vi "SimpleInterface.vi"() -> ()   [LabVIEW 2015]
panel:
  out "Amplitud\nP100":dbl
  out "N75":dbl
  out "P100":dbl
  out "N145":dbl
  out "Latencia \npromedio":dbl
  out "Resultado de las pruebas":cluster{dbl[], dbl[]}[](graph)
  in  "Cantidad de\nestímulos":dbl
  in  "Comenzar \nprueba":bool
  in  "Cantidad de \ncuadros":dbl
  in  "stop":bool
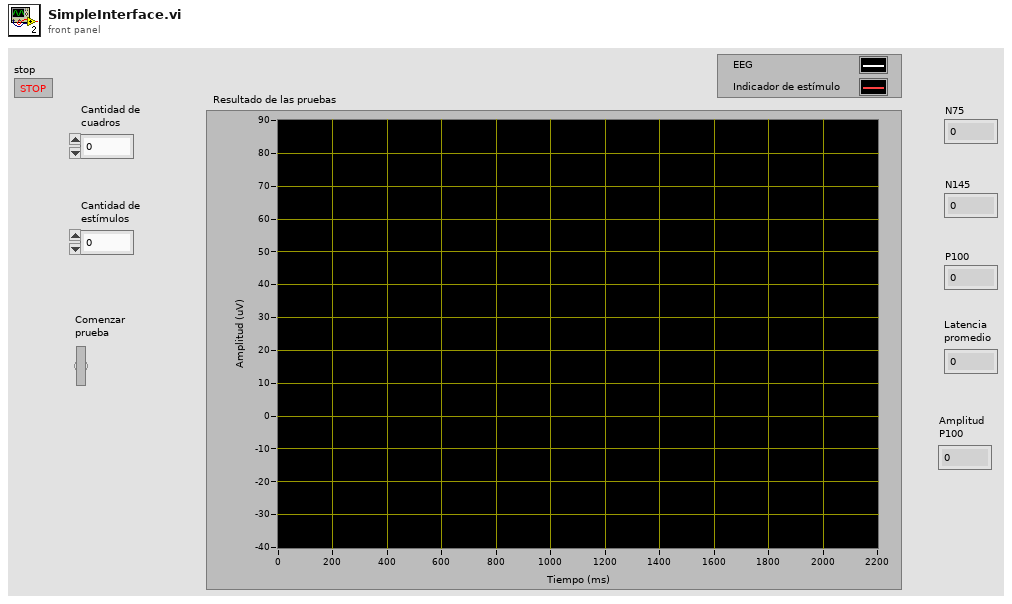
[diagram p1: front panel]
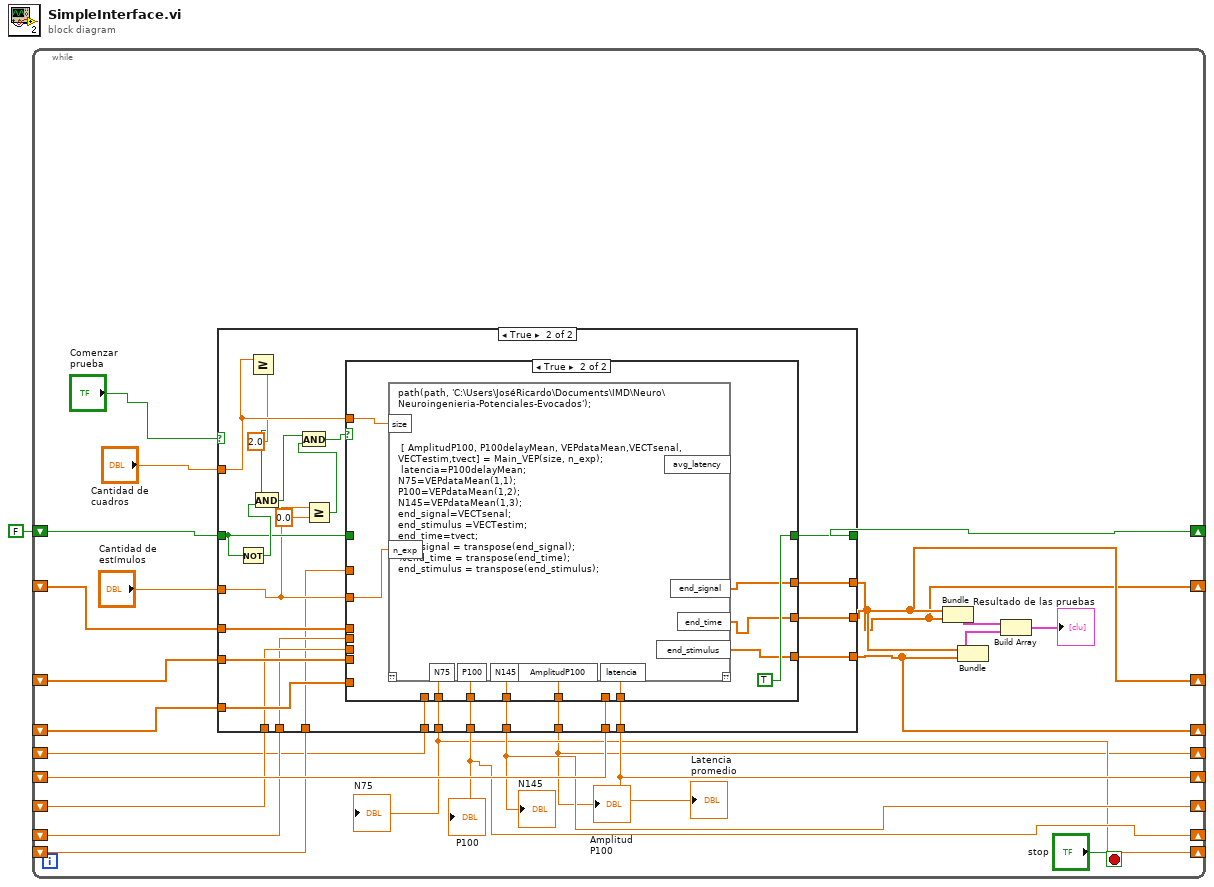
[diagram p0: block diagram]
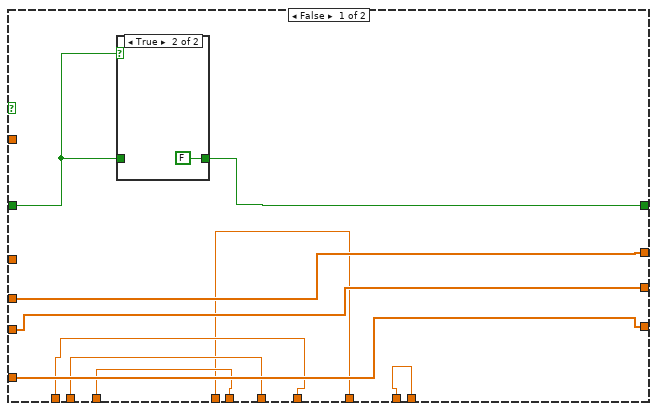
[diagram p2: hidden frame]
diagram:
  n1 = while {
    shift-right: [w25] -> _
    shift-left: FALSE -> [w23]
    shift-right: [w17] -> _
    shift-left: _ -> [w13]
    shift-right: [w16] -> _
    shift-left: _ -> [w14]
    shift-right: [w15] -> _
    shift-left: _ -> [w12]
    shift-right: [w11] -> _
    shift-left: _ -> [w10]
    shift-right: [w9] -> _
    shift-left: _ -> [w6]
    shift-right: [w8] -> _
    shift-left: _ -> [w5]
    shift-right: [w7] -> _
    shift-left: _ -> [w4]
    shift-right: [w3] -> _
    shift-left: _ -> [w2]
    stop <- "stop" stop-if-true
    n2 = case shown="True" "Comenzar \nprueba" {
      tunnel: [w36 w61] -> w25
      tunnel: "Cantidad de \ncuadros" -> [_ w65]
      tunnel: w23 -> [w35 w60]
      tunnel: "Cantidad de\nestímulos" -> [_ w59]
      tunnel: [w33 w54] -> w17
      tunnel: [w32 w53] -> w15
      tunnel: [w34 w52] -> w16
      tunnel: w14 -> [w34 w51]
      tunnel: w13 -> [w33 w50]
      tunnel: w12 -> [w32 w49]
      tunnel: [w31 w48] -> w11
      tunnel: w10 -> [w31 w47]
      tunnel: [w30 w46] -> w9
      tunnel: [w29 w45] -> w8
      tunnel: [w28 w44] -> w7
      tunnel: w6 -> [w30 w43]
      tunnel: w5 -> [w29 w42]
      tunnel: w4 -> [w28 w41]
      tunnel: [w27 w40] -> w3
      tunnel: w2 -> [w27 w39]
      frame False {
        n3 = case shown="True" w35 {
          tunnel: [w37 FALSE] -> w36
          tunnel: w35 -> [w37 _]
          frame False {
          }
          frame True {
          }
        }
      }
      frame True {
        n4 = Not(x=w60) -> (.not. x?=w63:bool)
        n5 = Greater Or Equal?(x=w65, y=2.0 ("x")) -> (x >= y?=w62:bool)
        n6 = And(x=w62, y=w63) -> (x .and. y?=w55:bool)
        n7 = Greater Or Equal?(x=w59, y=0.0) -> (x >= y?=w56:bool)
        n8 = And(x=w55, y=w56) -> (x .and. y?=w57:bool)
        n9 = case shown="True" w57 {
          tunnel: w65 -> [_ w85]
          tunnel: [w74 TRUE] -> w61
          tunnel: w60 -> [w74 _]
          tunnel: w59 -> [_ w83]
          tunnel: [w72 w82] -> w54
          tunnel: [w71 w81] -> w53
          tunnel: [w73 w80] -> w52
          tunnel: w51 -> [w73 _]
          tunnel: w50 -> [w72 _]
          tunnel: w49 -> [w71 _]
          tunnel: [w70 w79] -> w48
          tunnel: w47 -> [w70 _]
          tunnel: [w69 w78] -> w46
          tunnel: [w68 w77] -> w45
          tunnel: [w67 w76] -> w44
          tunnel: w43 -> [w69 _]
          tunnel: w42 -> [w68 _]
          tunnel: w41 -> [w67 _]
          tunnel: [w66 w75] -> w40
          tunnel: w39 -> [w66 _]
          frame False {
          }
          frame True {
            n10 = script code="path(path, 'C:\\Users\\JoséRicardo\\Documents\\IMD\\Neuro\\Neuroingenieria-Potenciales-Evocados');\n\n\n\n [ AmplitudP100, P100delayMean, VEPdataMean,VECTsenal, VECTestim,tvect] = Main_VEP(size, n_exp);\n latencia=P100delayMean;\nN75=VEPdataMean(1,1);\nP100=VEPdataMean(1,2);\nN145=VEPdataMean(1,3);\nend_signal=VECTsenal;\nend_stimulus =VECTestim;\nend_time=tvect;\nend_signal = transpose(end_signal);\n%end_time = transpose(end_time);\nend_stimulus = transpose(end_stimulus);"("size"=w85, "n_exp"=w83) -> ("end_signal"=w80:dbl[], "end_stimulus"=w81:dbl[], "end_time"=w82:dbl[], "latencia"=w79:dbl, "N75"=w76:dbl, "P100"=w77:dbl, "N145"=w78:dbl, "AmplitudP100"=w75:dbl)  [unwired: 1 in, 2 out]
          }
        }
      }
    }
    "Latencia \npromedio" <- w11
    "N145" <- w9
    "P100" <- w8
    "N75" <- w7
    "Amplitud\nP100" <- w3
    n11 = Bundle(w17, w16) -> (w19:cluster{dbl[], dbl[]})  [unwired: 1 in]
    n12 = Bundle(w17, w15) -> (w18:cluster{dbl[], dbl[]})  [unwired: 1 in]
    n13 = Build Array(w19, w18) -> (→"Resultado de las pruebas":cluster{dbl[], dbl[]}[])
  }
